vi "SRV_Generate Error.vi"(0 "status (T)":bool=TRUE, 1 "show call chain? (T)":bool=TRUE, 5 "code (42: generic error)":i32=42, 7 "Message":string, 9 "Pass Previous Error (T)":bool=TRUE, 11 "error in (no error)":errorcluster) -> (15 "error out":errorcluster)   [LabVIEW 2014]
doc: "Generates an error. Optionally puts the call chain in the error source if Call Chain is TRUE (default). The Error Code is 42 by default.\n\nAlso, it provides the option to overwrite a previous error with the new error (not recommended).\n\n\nAuthor: Mike Schultz"
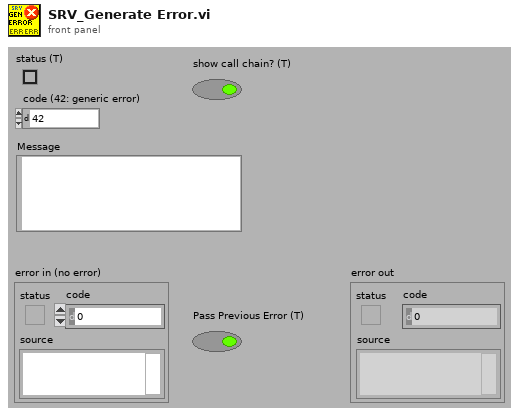
[diagram p1: front panel]
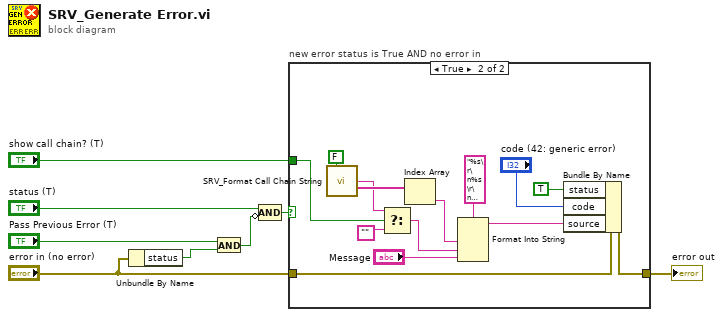
[diagram p0: block diagram]
diagram:
  n1 = Unbundle By Name("error in (no error)") -> ("status"=w5:bool)
  n2 = And(x="Pass Previous Error (T)", y=w5) -> (x .and. y?=w6:bool)
  n3 = Compound Arithmetic op=AND("status (T)", invert w6) -> (w7:bool)
  n4 = case "new error status is True AND no error in" shown="True" w7 {
    tunnel: "error in (no error)" -> [w9 w16]
    tunnel: [w9 w17] -> w3
    tunnel: "show call chain? (T)" -> [_ w13]
    frame False {
    }
    frame True {
      n5 = call "SRV_Format Call Chain String.vi"("Include This VI's Caller (T)"=FALSE) -> ("Formatted Call Chain String"=w12:string, "Trimmed Call Chain"=w14:string[])  [unwired: 13 in]
      n6 = Select(t=w12, s=w13, f="") -> (s? t:f=w11:string)
      n7 = Index Array(array=w14) -> (element=w19:string)  [unwired: 1 in]
      n8 = Format Into String(format string="%s\r\n%s\r\n%s", w19, w11, "Message") -> (resulting string=w23:string)  [unwired: 2 in, 1 out]
      n9 = Bundle By Name(cluster=w16, "status"=TRUE, "code"="code (42: generic error)", "source"=w23) -> (w17:errorcluster)
    }
  }
  "error out" <- w3
